vi "tx_dac.vi"(1 "fnco":dbl=190000000.0, 2 "fs":dbl=125000000.0, 3 "error in (no error)":errorcluster caption="错误输入（无错误）", 4 "fin":dbl[](array[numeric])=[218000000.0, 215000000.0, 220000000.0, 225000000.0, 230000000.0, 235000000.0, 240000000.0, 205000000.0, 200000000.0], 5 "开关":bool[](array[boolean])=[FALSE, TRUE, TRUE, FALSE, FALSE, FALSE, FALSE, TRUE, TRUE, FALSE], 6 "VISA resource name 2":refnum<visa-resource-name>="COM3" caption="VISA资源名称") -> (0 "error out":errorcluster={"status"=FALSE, "code"=1047, "source"=""})   [LabVIEW 2015]
uses:
  <vilib>/Instr/_visa.llb/VISA Configure Serial Port (Instr).vi
panel:
  out "连接的字符串":string
  out "VI":dbl[](array[numeric])
  out "Real":dbl
  out "CFG_RAM":bool
  out "TXPLL_INIT":bool
  out "DLL_MAN":bool
  out "EXT_CLK":bool
  in  "选项卡控件":enum32{"选项卡 1", "选项卡 2"}(tab)
  out "RF_out":dbl[](array[numeric])
  out "HQ":dbl[](array[numeric])
  out "HI":dbl[](array[numeric])
  out "VQ":dbl[](array[numeric])
  out "num_of_samples":dbl
  out "two":dbl
  out "predist":dbl
  out "one":dbl=1.0
  out "ten":dbl
  out "four":dbl
  out "three":dbl
  out "VISA resource name out":refnum<visa-resource-name>="COM3"
  # "EXT_CLK"
  # "TXPLL_INIT"
  # "ONE_TONE"
  # "TWO_TONE"
  # "THREE_TONE"
  # "FOUR_TONE"
  # "TEN_TONE"
  # "CFG_RAM"
  # "DLL_MAN"
  # "PREDIST"
  # "external clk&dll manul"
  # "external clk&dll auto"
  # "internal clk&dll manual"
  # "internal clk&dll auto"
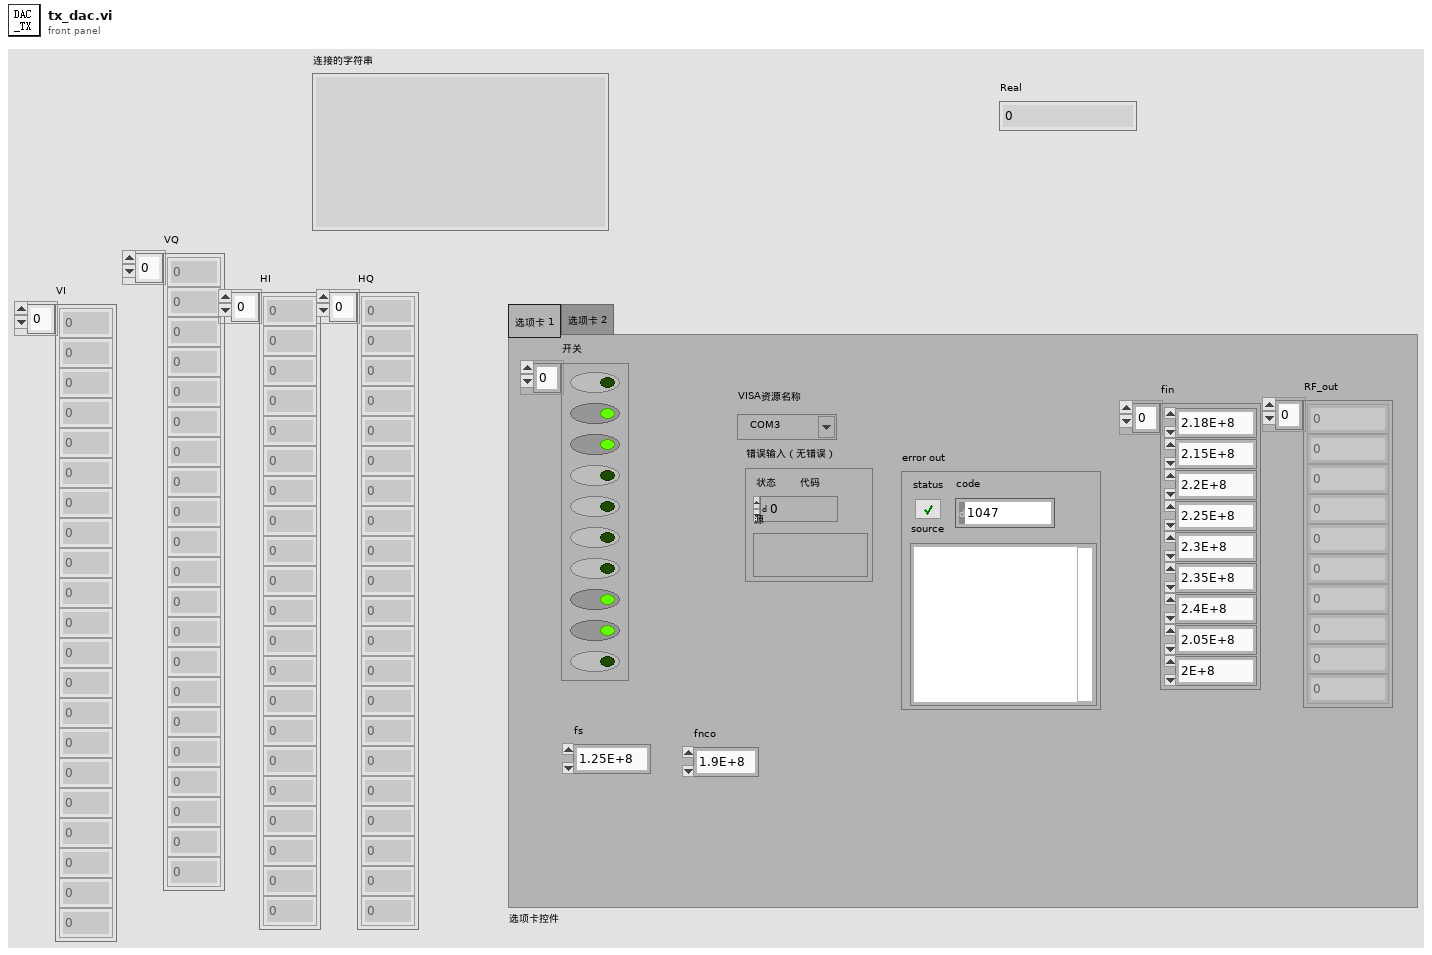
[diagram p1: front panel]
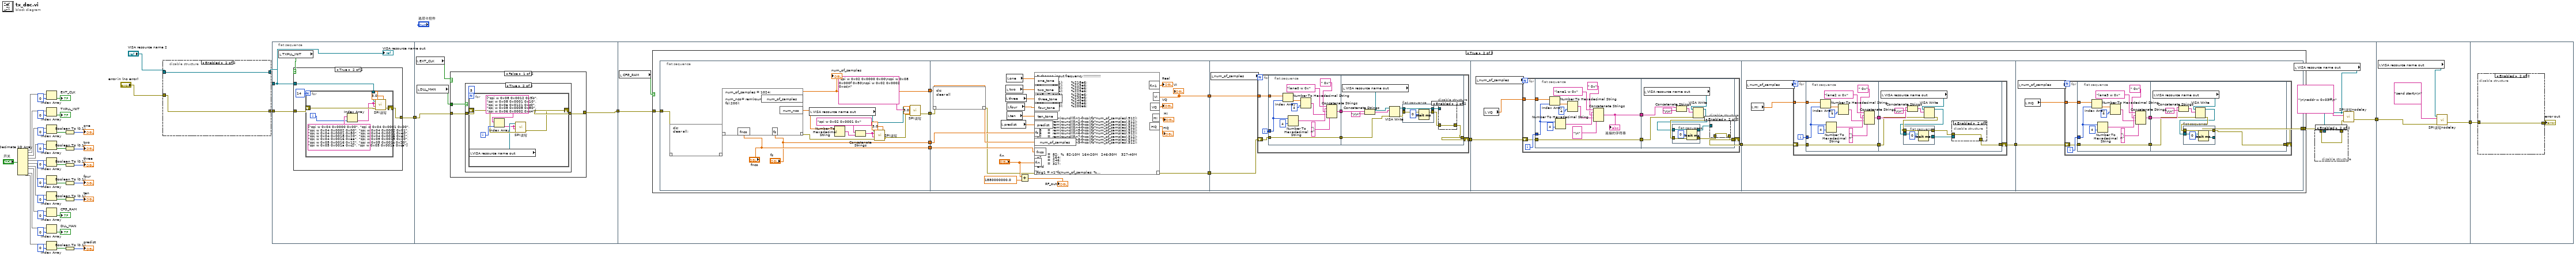
[diagram p0: block diagram]
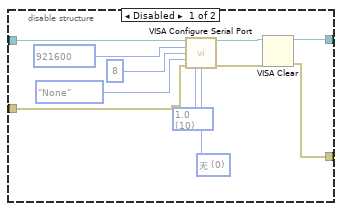
[diagram p2: hidden frame]
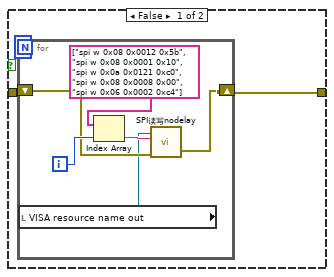
[diagram p4: hidden frame]
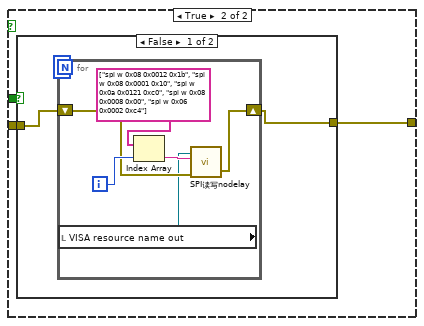
[diagram p5: hidden frame]
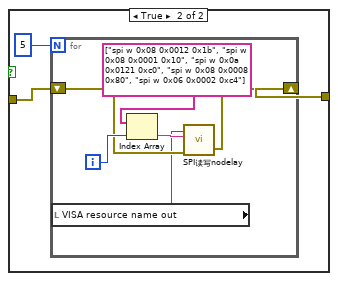
[diagram p6: hidden frame]
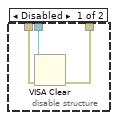
[diagram p7: hidden frame]
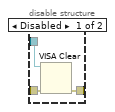
[diagram p9: hidden frame]
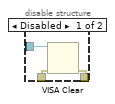
[diagram p10: hidden frame]
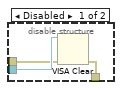
[diagram p11: hidden frame]
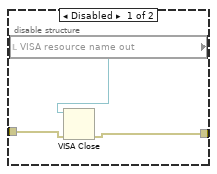
[diagram p12: hidden frame]
diagram:
  n1 = Decimate 1D Array("开关") -> (w32:bool[], w28:bool[], w25:bool[], w24:bool[], w22:bool[], w20:bool[], w18:bool[], w15:bool[], w12:bool[], w10:bool[])
  n2 = Index Array(array=w32, index=0 ("索引")) -> (element=→"EXT_CLK":bool)
  n3 = Index Array(array=w28, index=0 ("索引")) -> (element=→"TXPLL_INIT":bool)
  n4 = Index Array(array=w25, index=0 ("索引")) -> (element=w8:bool)
  n5 = Index Array(array=w24, index=0 ("索引")) -> (element=w7:bool)
  n6 = Index Array(array=w22, index=0 ("索引")) -> (element=w6:bool)
  n7 = Index Array(array=w20, index=0 ("索引")) -> (element=w5:bool)
  n8 = Index Array(array=w18, index=0 ("索引")) -> (element=w4:bool)
  n9 = Index Array(array=w15, index=0 ("索引")) -> (element=→"CFG_RAM":bool)
  n10 = Index Array(array=w12, index=0 ("索引")) -> (element=→"DLL_MAN":bool)
  n11 = Index Array(array=w10, index=0 ("索引")) -> (element=w3:bool)
  n12 = Boolean To (0,1)(Boolean=w8) -> (0, 1=→"one":i16)
  n13 = Boolean To (0,1)(Boolean=w7) -> (0, 1=→"two":i16)
  n14 = Boolean To (0,1)(Boolean=w6) -> (0, 1=→"three":i16)
  n15 = Boolean To (0,1)(Boolean=w5) -> (0, 1=→"four":i16)
  n16 = Boolean To (0,1)(Boolean=w4) -> (0, 1=→"ten":i16)
  n17 = Boolean To (0,1)(Boolean=w3) -> (0, 1=→"predist":i16)
  n18 = disable-structure shown="Enabled" {
    disable-tunnel: "VISA resource name 2" -> [w49 w58]
    disable-tunnel: "error in (no error)" -> [w48 w57]
    disable-tunnel: [w47 w58] -> w43
    disable-tunnel: [w46 w57] -> w42
    frame Disabled {
      w52 = u16 0 items=["无", "XON/XOFF", "RTS/CTS", "XON/XOFF & RTS/CTS", "DTR/DSR", "XON/XOFF & DTR/DSR"] ("flow control (0:none)")
      w53 = u16 10 items=["1.0"=10, "1.5"=15, "2.0"=20] ("stop bits (10: 1 bit)")
      n19 = call-poly "VISA Configure Serial Port"("VISA resource name"=w49, "baud rate (9600)"=u32 921600, "data bits (8)"=u16 8, "parity (0:none)"=enum16{"None", "Odd", "Even", "Mark", "Space"}."None", "error in (no error)"=w48, "stop bits (10: 1 bit)"=w53, "flow control (0:none)"=w52) -> ("VISA resource name out"=w51:refnum<visa-resource-name>, "error out"=w50:errorcluster)  [unwired: 7 in]
      n20 = VISA Clear(VISA resource name=w51, error in (no error)=w50) -> (VISA resource name out=w47:refnum<visa-resource-name>, error out=w46:errorcluster)
    }
    frame Enabled {
    }
  }
  n21 = flat-sequence {
    tunnel: w43 -> [w59]
    tunnel: w42 -> [w62]
    tunnel: [w61] -> w41
    tunnel: w41 -> [w78]
    tunnel: [w75] -> w2
    tunnel: [w125] -> w34
    tunnel: w2 -> [w127]
    tunnel: w34 -> [w331]
    tunnel: [w330] -> w1
    tunnel: w1 -> [w335]
    frame #0 {
      n22 = local read "TXPLL_INIT"() -> (w60:bool)
      n23 = case shown="True" w60 {
        tunnel: w59 -> [_ w67]
        tunnel: w62 -> [w63 w66]
        tunnel: [w63 w65] -> w61
        frame False {
        }
        frame True {
          n24 = for {
            N: 14 -> [_]
            tunnel: w67 -> [w69]
            shift-right: [w72] -> w65
            shift-left: w66 -> [w71]
            i -> [w73]
            n25 = Index Array(array=string[] ["spi w 0x04 0x0000 0x00", "spi w 0x04 0x0001 0x00", "spi w 0x04 0x0002 0x00", "spi w 0x04 0x0002 0x01", "spi w 0x04 0x0001 0x80", "spi w 0x04 0x0011 0xe0", "spi w 0x04 0x0018 0x20", "spi w 0x04 0x0016 0xe2", "spi w 0x04 0x0016 0xea", "spi w 0x05 0x0015 0x20", "spi w 0x05 0x0016 0x12", "spi w 0x05 0x001c 0x20", "spi w 0x05 0x001a 0xc2", "spi w 0x05 0x001a 0xca"], index=w73) -> (element=w70:string)
            n26 = call "SPI读写.vi"("DELAY"=3.0, "error in (no error)"=w71, "从芯片读数据"=w70, "往芯片写数据"=w70, "VISA resource name"=w69) -> ("error out"=w72:errorcluster)  [unwired: 1 out]
          }
        }
      }
      "VISA resource name out" <- w59
    }
    frame #1 {
      n27 = local read "EXT_CLK"() -> (w77:bool)
      n28 = local read "DLL_MAN"() -> (w76:bool)
      n29 = case shown="False" w77 {
        tunnel: w76 -> [w81 w102]
        tunnel: [w80 w101] -> w75
        tunnel: w78 -> [w79 w100]
        frame False {
          n30 = case shown="True" w81 {
            tunnel: [w83 w91] -> w80
            tunnel: w79 -> [w84 w92]
            frame False {
              n31 = for {
                N: 5 -> [_]
                shift-right: [w86] -> w83
                shift-left: w84 -> [w87]
                i -> [w90]
                n32 = local read "VISA resource name out"() -> (w85:refnum<visa-resource-name>)
                n33 = Index Array(array=string[] ["spi w 0x08 0x0012 0x5b", "spi w 0x08 0x0001 0x10", "spi w 0x0a 0x0121 0xc0", "spi w 0x08 0x0008 0x00", "spi w 0x06 0x0002 0xc4"], index=w90) -> (element=w88:string)
                n34 = call "SPI读写nodelay.vi"("error in (no error)"=w87, "往芯片写数据"=w88, "VISA resource name"=w85) -> ("error out"=w86:errorcluster)  [unwired: 1 in, 1 out]
              }
            }
            frame True {
              n35 = for {
                N: 5 -> [_]
                shift-right: [w97] -> w91
                shift-left: w92 -> [w96]
                i -> [w99]
                n36 = local read "VISA resource name out"() -> (w95:refnum<visa-resource-name>)
                n37 = Index Array(array=string[] ["spi w 0x08 0x0012 0x5b", "spi w 0x08 0x0001 0x10", "spi w 0x0a 0x0121 0xc0", "spi w 0x08 0x0008 0x80", "spi w 0x06 0x0002 0xc4"], index=w99) -> (element=w94:string)
                n38 = call "SPI读写.vi"("error in (no error)"=w96, "从芯片读数据"=w94, "往芯片写数据"=w94, "VISA resource name"=w95) -> ("error out"=w97:errorcluster)  [unwired: 1 in, 1 out]
              }
            }
          }
        }
        frame True {
          n39 = case shown="False" w102 {
            tunnel: [w104 w113] -> w101
            tunnel: w100 -> [w105 w114]
            frame False {
              n40 = for {
                N: 5 -> [_]
                shift-right: [w107] -> w104
                shift-left: w105 -> [w108]
                i -> [w111]
                n41 = local read "VISA resource name out"() -> (w106:refnum<visa-resource-name>)
                n42 = Index Array(array=string[] ["spi w 0x08 0x0012 0x1b", "spi w 0x08 0x0001 0x10", "spi w 0x0a 0x0121 0xc0", "spi w 0x08 0x0008 0x00", "spi w 0x06 0x0002 0xc4"], index=w111) -> (element=w109:string)
                n43 = call "SPI读写nodelay.vi"("error in (no error)"=w108, "往芯片写数据"=w109, "VISA resource name"=w106) -> ("error out"=w107:errorcluster)  [unwired: 1 in, 1 out]
              }
            }
            frame True {
              n44 = for {
                N: 5 -> [_]
                shift-right: [w116] -> w113
                shift-left: w114 -> [w117]
                i -> [w120]
                n45 = local read "VISA resource name out"() -> (w115:refnum<visa-resource-name>)
                n46 = Index Array(array=string[] ["spi w 0x08 0x0012 0x1b", "spi w 0x08 0x0001 0x10", "spi w 0x0a 0x0121 0xc0", "spi w 0x08 0x0008 0x80", "spi w 0x06 0x0002 0xc4"], index=w120) -> (element=w118:string)
                n47 = call "SPI读写nodelay.vi"("error in (no error)"=w117, "往芯片写数据"=w118, "VISA resource name"=w115) -> ("error out"=w116:errorcluster)  [unwired: 1 in, 1 out]
              }
            }
          }
        }
      }
    }
    frame #2 {
      n48 = local read "CFG_RAM"() -> (w124:bool)
      n49 = case shown="True" w124 {
        tunnel: w127 -> [w132 w143]
        tunnel: [w132 w138] -> w122
        frame False {
        }
        frame True {
          n50 = flat-sequence {
            tunnel: w143 -> [w154]
            tunnel: [w151] -> w142
            tunnel: [w156] -> w141
            tunnel: ["fs"] -> w134
            tunnel: ["fnco"] -> w133
            tunnel: w142 -> [w161]
            tunnel: w141 -> [w179]
            tunnel: [w172] -> w140
            tunnel: [w171] -> w139
            tunnel: w134 -> [w167]
            tunnel: w133 -> [w166]
            tunnel: w140 -> [w181]
            tunnel: w139 -> [w182]
            tunnel: [w180] -> w135
            tunnel: [w220] -> w136
            tunnel: w135 -> [w219]
            tunnel: [w259] -> w137
            tunnel: w136 -> [w258]
            tunnel: [w298] -> w138
            tunnel: w137 -> [w297]
            frame #0 {
              w150 = "spi w 0x02 0x0000 0x00\nspi w 0x08 0x000f 0x80\nspi w 0x02 0x0002 0xcc\n" ("往芯片写数据")
              n51 = script code="clc;\nclear all;"("??"=w154) -> ("??"=w153:errorcluster)
              n52 = script code="num_of_samples = 1024;\n\nnum_nco= rem(round(fnco/5e6*125e6/fs),200);"("??"=w153, "fnco"="fnco", "fs"="fs") -> ("??"=w145:errorcluster, "num_of_samples"=w156:dbl, "num_nco"=w157:dbl)
              "num_of_samples" <- w156
              n53 = local read "VISA resource name out"() -> (w147:refnum<visa-resource-name>)
              n54 = Number To Hexadecimal String(2:w157) -> (0:w159:string)  [unwired: 1 in]
              n55 = Concatenate Strings("spi w 0x02 0x0001 0x", w159) -> (w148:string)
              n56 = call "SPI读写.vi"("DELAY"=3.0, "error in (no error)"=w145, "从芯片读数据"=w148, "往芯片写数据"=w148, "VISA resource name"=w147) -> ("error out"=w146:errorcluster)  [unwired: 1 out]
              n57 = call "SPI读写.vi"("DELAY"=3.0, "error in (no error)"=w146, "从芯片读数据"=w150, "往芯片写数据"=w150, "VISA resource name"=w147) -> ("error out"=w151:errorcluster)  [unwired: 1 out]
            }
            frame #1 {
              n58 = script code="clc;\nclear all"("??"=w161) -> ("??"=w160:errorcluster)
              n59 = local read "predist"() -> (w173:dbl)
              n60 = local read "three"() -> (w176:dbl)
              n61 = local read "two"() -> (w177:dbl)
              n62 = local read "one"() -> (w178:dbl)
              n63 = local read "four"() -> (w175:dbl)
              n64 = local read "ten"() -> (w174:dbl)
              n65 = Add(x="fin", y=1880000000.0) -> (x+y=→"RF_out":dbl[])
              n66 = script code="%change input frequency!!!!!!!!!!!!!!!\n\nfin1   =  fin(1);       %218e6;\nfin2   =  fin(2);       %215e6;\nfin3   =  fin(3);       %220e6;\nfin4   =  fin(4);       %225e6;\nfin5   =  fin(5);       %230e6;\nfin6   =  fin(6);       %235e6;\nfin7   =  fin(7);       %240e6;\nfin8   =  fin(8);       %205e6;\nfin9   =  fin(9);       %200e6;\n\n\n\nn1     =  rem(round((fin1-fnco)/fs*num_of_samples),512);\nn2     =  rem(round((fin2-fnco)/fs*num_of_samples),512);\nn3     =  rem(round((fin3-fnco)/fs*num_of_samples),512);\nn4     =  rem(round((fin4-fnco)/fs*num_of_samples),512);\nn5     =  rem(round((fin5-fnco)/fs*num_of_samples),512);\nn6     =  rem(round((fin6-fnco)/fs*num_of_samples),512);\nn7     =  rem(round((fin7-fnco)/fs*num_of_samples),512);\nn8     =  rem(round((fin8-fnco)/fs*num_of_samples),512);\nn9     =  rem(round((fin9-fnco)/fs*num_of_samples),512);\n\n\nif 0\nn1     =  82;  %  82-10M  164-20M   246-30M    327-40M\nn2     =  164;\nn3     =  246;\nn4     =  327;\nend\n\nfsig1 = n1*fs/num_of_samples; % \nfsig2 = n2*fs/num_of_samples;  % \nfsig3 = n3*fs/num_of_samples;\nfsig4 = n4*fs/num_of_samples;\nfsig5 = n5*fs/num_of_samples;\nfsig6 = n6*fs/num_of_samples;\nfsig7 = n7*fs/num_of_samples;\nfsig8 = n8*fs/num_of_samples;\nfsig9 = n9*fs/num_of_samples;\n\n\n\nbits = 14;\namp  = -1;\n\n\nif one_tone\n    amp = -1;   %%% dBFs default:-1\nend\nif two_tone\n    amp = -10.2;   %%% dBFs default:-1\nend\nif three_tone\n    amp = -9.2;   %%% dBFs default:-1\nend\nif four_tone\n    amp = -16;   %%% dBFs default:-1\nend\n\nf1 = (0:1:num_of_samples-1)*fsig1/fs*2*pi;\nf2 = (0:1:num_of_samples-1)*fsig2/fs*2*pi;\nf3 = (0:1:num_of_samples-1)*fsig3/fs*2*pi;\nf4 = (0:1:num_of_samples-1)*fsig4/fs*2*pi;\nf5 = (0:1:num_of_samples-1)*fsig5/fs*2*pi;\nf6 = (0:1:num_of_samples-1)*fsig6/fs*2*pi;\nf7 = (0:1:num_of_samples-1)*fsig7/fs*2*pi;\nf8 = (0:1:num_of_samples-1)*fsig8/fs*2*pi;\nf9 = (0:1:num_of_samples-1)*fsig9/fs*2*pi;\n\nf1_dly = ((0:1:num_of_samples-1)+0.74)*fsig1/fs*2*pi;\nf2_dly = ((0:1:num_of_samples-1)+0.59)*fsig2/fs*2*pi;\nf3_dly = ((0:1:num_of_samples-1)+0.74)*fsig3/fs*2*pi;\nf4_dly = ((0:1:num_of_samples-1)+0.59)*fsig4/fs*2*pi;\n\n\n\namp_dig = round(2^(bits-1)*10^(amp/20));\namp_dig2 = round(2^(bits-1)*10^((amp-0)/20));\namp_dig3 = round(2^(bits-1)*10^((amp-0)/20));\namp_dig4 = round(2^(bits-1)*10^((amp-0)/20));\n\n\n if(one_tone)\n     LHP_I = round(amp_dig*(cos(f1)));\n     LHP_Q = round(amp_dig*(cos(f1)));\n     RHP_I = round(amp_dig*(sin(f1)));\n     RHP_Q = round(amp_dig*(sin(f1)));\n     \n     \n          \n elseif(two_tone)\n     LHP_I = round(amp_dig*(cos(f1))+amp_dig2*(cos(f2)));\n     LHP_Q = round(amp_dig*(cos(f1))+amp_dig2*(cos(f2)));\n     RHP_I = round(amp_dig*(sin(f1))+amp_dig2*(sin(f2)));\n     RHP_Q = round(amp_dig*(sin(f1))+amp_dig2*(sin(f2)));\n \n     \n     \n elseif(three_tone)\n     LHP_I = round(amp_dig*(cos(f1))+amp_dig2*(cos(f2))+amp_dig3*(cos(f3)));\n     LHP_Q = round(amp_dig*(sin(f2))+amp_dig2*(cos(f2))+amp_dig3*(cos(f3)));\n     RHP_I = round(amp_dig*(sin(f3))+amp_dig2*(sin(f2))+amp_dig3*(sin(f3)));\n     RHP_Q = round(amp_dig*(sin(f4))+amp_dig2*(sin(f2))+amp_dig3*(sin(f3)));\n     \n elseif(four_tone)\n     LHP_I = round(amp_dig*(cos(f1))+amp_dig2*(cos(f2))+amp_dig3*(cos(f3))+amp_dig4*(cos(f4)));\n     LHP_Q = round(amp_dig*(cos(f1))+amp_dig2*(cos(f2))+amp_dig3*(cos(f3))+amp_dig4*(cos(f4)));\n     RHP_I = round(amp_dig*(sin(f1))+amp_dig2*(sin(f2))+amp_dig3*(sin(f3))+amp_dig4*(sin(f4)));\n     RHP_Q = round(amp_dig*(sin(f1))+amp_dig2*(sin(f2))+amp_dig3*(sin(f3))+amp_dig4*(sin(f4)));\n  \n         \n elseif(ten_tone)  \n      LHP_I = round(amp_dig*(cos(f1))+amp_dig2*(cos(f2))+amp_dig3*(cos(f3))+amp_dig4*(cos(f4))+amp_dig4*(cos(f5))+amp_dig4*(cos(f6))+amp_dig4*(cos(f7))+amp_dig4*(cos(f8))+amp_dig4*(cos(f9)));\n      LHP_Q = round(amp_dig*(cos(f1))+amp_dig2*(cos(f2))+amp_dig3*(cos(f3))+amp_dig4*(cos(f4))+amp_dig4*(cos(f5))+amp_dig4*(cos(f6))+amp_dig4*(cos(f7))+amp_dig4*(cos(f8))+amp_dig4*(cos(f9)));\n      RHP_I = round(amp_dig*(cos(f1))+amp_dig2*(cos(f2))+amp_dig3*(cos(f3))+amp_dig4*(cos(f4))+amp_dig4*(cos(f5))+amp_dig4*(cos(f6))+amp_dig4*(cos(f7))+amp_dig4*(cos(f8))+amp_dig4*(cos(f9)));\n      RHP_Q = round(amp_dig*(cos(f1))+amp_dig2*(cos(f2))+amp_dig3*(cos(f3))+amp_dig4*(cos(f4))+amp_dig4*(cos(f5))+amp_dig4*(cos(f6))+amp_dig4*(cos(f7))+amp_dig4*(cos(f8))+amp_dig4*(cos(f9)));\n     \n\n else\n     LHP_I = round(amp_dig*(cos(f1)));\n     LHP_Q = round(amp_dig*(cos(f2)));\n     RHP_I = round(amp_dig*(sin(f3)));\n     RHP_Q = round(amp_dig*(sin(f4)));\n\n end\n \n  VI = (LHP_I + RHP_I)/2; \n  VQ = (RHP_Q - LHP_Q)/2;\n  HI = (LHP_I + RHP_I)/2; \n  HQ = (RHP_Q - LHP_Q)/2;\n  \n  if(predist)\n      k_final1 = -19.58;\n      k_final2 = -19.98;   \n      amp_final1 = round(2^(bits-1)*10^(k_final1/20));\n      amp_final2 = round(2^(bits-1)*10^(k_final2/20));  \n  \n      if(two_tone)\n          LHP_I_dly = round(amp_dig*(cos(f1_dly))+amp_dig2*(cos(f2_dly)));\n          LHP_Q_dly = round(amp_dig*(cos(f1_dly))+amp_dig2*(cos(f2_dly)));\n          RHP_I_dly = round(amp_dig*(sin(f1_dly))+amp_dig2*(sin(f2_dly)));\n          RHP_Q_dly = round(amp_dig*(sin(f1_dly))+amp_dig2*(sin(f2_dly)));    \n      elseif(four_tone)\n          LHP_I_dly = round(amp_dig*(cos(f1_dly))+amp_dig2*(cos(f2_dly))+amp_dig3*(cos(f3_dly))+amp_dig4*(cos(f4_dly)));\n          LHP_Q_dly = round(amp_dig*(cos(f1_dly))+amp_dig2*(cos(f2_dly))+amp_dig3*(cos(f3_dly))+amp_dig4*(cos(f4_dly)));\n          RHP_I_dly = round(amp_dig*(sin(f1_dly))+amp_dig2*(sin(f2_dly))+amp_dig3*(sin(f3_dly))+amp_dig4*(sin(f4_dly)));\n          RHP_Q_dly = round(amp_dig*(sin(f1_dly))+amp_dig2*(sin(f2_dly))+amp_dig3*(sin(f3_dly))+amp_dig4*(sin(f4_dly)));  \n      end\n  \n      VI_dly = (LHP_I_dly + RHP_I_dly)/2; \n      VQ_dly = (RHP_Q_dly - LHP_Q_dly)/2;\n      HI_dly = (LHP_I_dly + RHP_I_dly)/2; \n      HQ_dly = (RHP_Q_dly - LHP_Q_dly)/2;  \n   \n      VI = VI + round(amp_final1*(VI_dly/8192).^3) ;\n      VQ = VQ + round(amp_final2*(VQ_dly/8192).^3) ;\n      HI = HI + round(amp_final1*(HI_dly/8192).^3);\n      HQ = HQ + round(amp_final2*(HQ_dly/8192).^3) ;\n  end\n    \n\n  VI = round(VI); \n  VQ = round(VQ); \n  HI = round(HI); \n  HQ = round(HQ); \n  \n  VI(find(VI<0))=VI(find(VI<0))+16384;\n  VQ(find(VQ<0))=VQ(find(VQ<0))+16384;\n  HI(find(HI<0))=HI(find(HI<0))+16384;\n  HQ(find(HQ<0))=HQ(find(HQ<0))+16384;"("??"=w160, "one_tone"=w178, "two_tone"=w177, "three_tone"=w176, "four_tone"=w175, "ten_tone"=w174, "predist"=w173, "fs"=w167, "num_of_samples"=w179, "fnco"=w166, "fin"="fin") -> ("??"=w172:errorcluster, "VI"=w171:dbl[], "VQ"=→"VQ":dbl[], "HI"=→"HI":dbl[], "HQ"=→"HQ":dbl[], "fin1"=→"Real":dbl)
              "VI" <- w171
            }
            frame #2 {
              n67 = local read "num_of_samples"() -> (w183:dbl)
              n68 = for {
                N: w183 -> [_]
                tunnel: w182 -> [w188]
                shift-right: [w184] -> w180
                shift-left: w181 -> [w185]
                i -> [w189]
                n69 = flat-sequence {
                  tunnel: w189 -> [w200]
                  tunnel: w188 -> [w199]
                  tunnel: [w191] -> w187
                  tunnel: [w190] -> w186
                  tunnel: w185 -> [w190]
                  tunnel: w187 -> [w210]
                  tunnel: w186 -> [w207]
                  tunnel: [w202] -> w184
                  frame #0 {
                    n70 = Index Array(array=w199, index=w200) -> (element=w197:dbl)
                    n71 = Number To Hexadecimal String(1:i16 4 ("宽度(-)"), 2:w200) -> (0:w196:string)
                    n72 = Number To Hexadecimal String(1:i16 4 ("宽度(-)"), 2:w197) -> (0:w194:string)
                    n73 = Concatenate Strings("lane0 w 0x" ("字符串"), w196, " 0x" ("字符串"), w194, "\n" ("字符串")) -> (w191:string)
                  }
                  frame #1 {
                    n74 = local read "VISA resource name out"() -> (w211:refnum<visa-resource-name>)
                    n75 = Concatenate Strings(w210, "\r\n") -> (w208:string)
                    n76 = VISA Write(VISA resource name=w211, write buffer=w208, error in (no error)=w207) -> (VISA resource name out=w206:refnum<visa-resource-name>, error out=w205:errorcluster)  [unwired: 1 out]
                    n77 = flat-sequence {
                      tunnel: [w217] -> w204
                      tunnel: w206 -> [w217]
                      tunnel: [w216] -> w203
                      tunnel: w205 -> [w216]
                      frame #0 {
                        n78 = Wait (ms)(milliseconds to wait=u32 0 ("等待时间（毫秒）")) -> ()  [unwired: 1 out]
                      }
                    }
                    n79 = disable-structure shown="Enabled" {
                      disable-tunnel: w204 -> [w214 _]
                      disable-tunnel: w203 -> [w213 w215]
                      disable-tunnel: [w212 w215] -> w202
                      frame Disabled {
                        n80 = VISA Clear(VISA resource name=w214, error in (no error)=w213) -> (error out=w212:errorcluster)  [unwired: 1 out]
                      }
                      frame Enabled {
                      }
                    }
                  }
                }
              }
            }
            frame #3 {
              n81 = local read "num_of_samples"() -> (w222:dbl)
              n82 = local read "VQ"() -> (w221:dbl[])
              n83 = for {
                N: w222 -> [_]
                tunnel: w221 -> [w227]
                shift-right: [w223] -> w220
                shift-left: w219 -> [w224]
                i -> [w228]
                n84 = flat-sequence {
                  tunnel: w228 -> [w239]
                  tunnel: w227 -> [w238]
                  tunnel: [w230] -> w226
                  tunnel: [w229] -> w225
                  tunnel: w224 -> [w229]
                  tunnel: w226 -> [w250]
                  tunnel: w225 -> [w246]
                  tunnel: [w241] -> w223
                  frame #0 {
                    n85 = Index Array(array=w238, index=w239) -> (element=w236:dbl)
                    n86 = Number To Hexadecimal String(1:i16 4 ("宽度(-)"), 2:w239) -> (0:w235:string)
                    n87 = Number To Hexadecimal String(1:i16 4 ("宽度(-)"), 2:w236) -> (0:w233:string)
                    n88 = Concatenate Strings("lane1 w 0x" ("字符串"), w235, " 0x" ("字符串"), w233, "\n" ("字符串")) -> (w230:string)
                    "连接的字符串" <- w230
                  }
                  frame #1 {
                    n89 = local read "VISA resource name out"() -> (w247:refnum<visa-resource-name>)
                    n90 = flat-sequence {
                      tunnel: [w256] -> w242
                      tunnel: w245 -> [w256]
                      tunnel: [w255] -> w243
                      tunnel: w244 -> [w255]
                      frame #0 {
                        n91 = Wait (ms)(milliseconds to wait=u32 0 ("等待时间（毫秒）")) -> ()  [unwired: 1 out]
                      }
                    }
                    n92 = Concatenate Strings(w250, "\r\n") -> (w248:string)
                    n93 = VISA Write(VISA resource name=w247, write buffer=w248, error in (no error)=w246) -> (VISA resource name out=w244:refnum<visa-resource-name>, error out=w245:errorcluster)  [unwired: 1 out]
                    n94 = disable-structure shown="Enabled" {
                      disable-tunnel: w243 -> [w253 _]
                      disable-tunnel: w242 -> [w252 w254]
                      disable-tunnel: [w251 w254] -> w241
                      frame Disabled {
                        n95 = VISA Clear(VISA resource name=w253, error in (no error)=w252) -> (error out=w251:errorcluster)  [unwired: 1 out]
                      }
                      frame Enabled {
                      }
                    }
                  }
                }
              }
            }
            frame #4 {
              n96 = local read "num_of_samples"() -> (w261:dbl)
              n97 = local read "HI"() -> (w260:dbl[])
              n98 = for {
                N: w261 -> [_]
                tunnel: w260 -> [w266]
                shift-right: [w262] -> w259
                shift-left: w258 -> [w263]
                i -> [w267]
                n99 = flat-sequence {
                  tunnel: w267 -> [w278]
                  tunnel: w266 -> [w277]
                  tunnel: [w269] -> w265
                  tunnel: [w268] -> w264
                  tunnel: w263 -> [w268]
                  tunnel: w265 -> [w287]
                  tunnel: w264 -> [w286]
                  tunnel: [w280] -> w262
                  frame #0 {
                    n100 = Index Array(array=w277, index=w278) -> (element=w275:dbl)
                    n101 = Number To Hexadecimal String(1:i16 4 ("宽度(-)"), 2:w278) -> (0:w274:string)
                    n102 = Number To Hexadecimal String(1:i16 4 ("宽度(-)"), 2:w275) -> (0:w272:string)
                    n103 = Concatenate Strings("lane2 w 0x" ("字符串"), w274, " 0x" ("字符串"), w272, "\n" ("字符串")) -> (w269:string)
                  }
                  frame #1 {
                    n104 = local read "VISA resource name out"() -> (w285:refnum<visa-resource-name>)
                    n105 = flat-sequence {
                      tunnel: [w295] -> w281
                      tunnel: w284 -> [w295]
                      tunnel: [w294] -> w282
                      tunnel: w283 -> [w294]
                      frame #0 {
                        n106 = Wait (ms)(milliseconds to wait=u32 0 ("等待时间（毫秒）")) -> ()  [unwired: 1 out]
                      }
                    }
                    n107 = Concatenate Strings(w287, "\r\n") -> (w289:string)
                    n108 = VISA Write(VISA resource name=w285, write buffer=w289, error in (no error)=w286) -> (VISA resource name out=w283:refnum<visa-resource-name>, error out=w284:errorcluster)  [unwired: 1 out]
                    n109 = disable-structure shown="Enabled" {
                      disable-tunnel: w282 -> [w292 _]
                      disable-tunnel: w281 -> [w291 w293]
                      disable-tunnel: [w290 w293] -> w280
                      frame Disabled {
                        n110 = VISA Clear(VISA resource name=w292, error in (no error)=w291) -> (error out=w290:errorcluster)  [unwired: 1 out]
                      }
                      frame Enabled {
                      }
                    }
                  }
                }
              }
            }
            frame #5 {
              n111 = local read "num_of_samples"() -> (w300:dbl)
              n112 = local read "HQ"() -> (w299:dbl[])
              n113 = for {
                N: w300 -> [_]
                tunnel: w299 -> [w305]
                shift-right: [w301] -> w298
                shift-left: w297 -> [w302]
                i -> [w306]
                n114 = flat-sequence {
                  tunnel: w306 -> [w317]
                  tunnel: w305 -> [w316]
                  tunnel: [w308] -> w304
                  tunnel: [w307] -> w303
                  tunnel: w302 -> [w307]
                  tunnel: w304 -> [w324]
                  tunnel: w303 -> [w322]
                  tunnel: [w319] -> w301
                  frame #0 {
                    n115 = Index Array(array=w316, index=w317) -> (element=w314:dbl)
                    n116 = Number To Hexadecimal String(1:i16 4 ("宽度(-)"), 2:w317) -> (0:w313:string)
                    n117 = Number To Hexadecimal String(1:i16 4 ("宽度(-)"), 2:w314) -> (0:w311:string)
                    n118 = Concatenate Strings("lane3 w 0x" ("字符串"), w313, " 0x" ("字符串"), w311, "\n" ("字符串")) -> (w308:string)
                  }
                  frame #1 {
                    n119 = local read "VISA resource name out"() -> (w323:refnum<visa-resource-name>)
                    n120 = Concatenate Strings(w324, "\r\n") -> (w325:string)
                    n121 = flat-sequence {
                      tunnel: [w328] -> w319
                      tunnel: w321 -> [w328]
                      tunnel: [w327] -> _
                      tunnel: w320 -> [w327]
                      frame #0 {
                        n122 = Wait (ms)(milliseconds to wait=u32 0 ("等待时间（毫秒）")) -> ()  [unwired: 1 out]
                      }
                    }
                    n123 = VISA Write(VISA resource name=w323, write buffer=w325, error in (no error)=w322) -> (VISA resource name out=w320:refnum<visa-resource-name>, error out=w321:errorcluster)  [unwired: 1 out]
                  }
                }
              }
            }
          }
        }
      }
      n124 = local read "VISA resource name out"() -> (w121:refnum<visa-resource-name>)
      n125 = disable-structure shown="Enabled" {
        disable-tunnel: [w130 w131] -> w123
        disable-tunnel: w122 -> [w129 w131]
        disable-tunnel: w121 -> [w128 _]
        frame Disabled {
          n126 = VISA Clear(VISA resource name=w128, error in (no error)=w129) -> (error out=w130:errorcluster)  [unwired: 1 out]
        }
        frame Enabled {
        }
      }
      n127 = call "SPI读写nodelay.vi"("error in (no error)"=w123, "往芯片写数据"="\n\naddr w 0x03ff\n", "VISA resource name"=w121) -> ("error out"=w125:errorcluster)  [unwired: 1 in, 1 out]
    }
    frame #3 {
      n128 = local read "VISA resource name out"() -> (w332:refnum<visa-resource-name>)
      n129 = call "SPI读写nodelay.vi"("error in (no error)"=w331, "往芯片写数据"="send start\n\n", "VISA resource name"=w332) -> ("error out"=w330:errorcluster)  [unwired: 1 in, 1 out]
    }
    frame #4 {
      n130 = disable-structure shown="Enabled" {
        disable-tunnel: w335 -> [w338 w339]
        disable-tunnel: [w337 w339] -> w334
        frame Disabled {
          n131 = local read "VISA resource name out"() -> (w336:refnum<visa-resource-name>)
          n132 = VISA Close(VISA resource name=w336, error in (no error)=w338) -> (error out=w337:errorcluster)
        }
        frame Enabled {
        }
      }
      "error out" <- w334
    }
  }
